vi "Get Scan area.vi"(7 "Inspection data":T1, 8 "error in (no error)":errorcluster, 11 "Programming Data":T12) -> (0 "error out":errorcluster, 2 "Panel size Y":dbl, 3 "Panel Size X":dbl)   [LabVIEW 2013, in "Manipulate IPF.lvlib"]
uses:
  Manipulate IPF.lvlib
  type_def/files.ctl
  3013/code/Modules/Inspection/Data/Panel_class/type_def/Config File data.ctl
  3013/code/Modules/Inspection/type_def/Pos and Rot.ctl
  3013/code/Modules/Inspection/Data/PCB_class/type_def/PCB Params.ctl
  3013/code/Modules/Inspection/Data/Panel_class/type_def/BarCode Params.ctl
  3013/code/Modules/Barcode Reader/type_def/id.ctl
  3013/code/Modules/GUI/GUI_5/subPanels/edit/type_def/data.ctl
  3013/code/Modules/Configuration/type_def/Scan Params.ctl
  3013/code/Modules/Configuration/type_def/Profile Resolution.ctl
  3013/code/Modules/Preprocess Data/type_def/direction.ctl
  3013/code/Modules/Inspection/Data/Panel_class/type_def/inspection data.ctl
  3013/code/Modules/Inspection/type_def/Range Limits.ctl
  type_def/Initial scan size increase.ctl
  <vilib>/Analysis/coordinate.llb/2D Cartesian Coordinate Rotation (Array).vi
  <vilib>/Analysis/coordinate.llb/2D Cartesian Coordinate Shift (Array).vi
  <vilib>/Utility/file.llb/Read From Spreadsheet File (DBL).vi
  <vilib>/Analysis/NI_AALPro.lvlib
  3013/code/Modules/Inspection/Inspection.lvlib
  3013/code/Modules/Inspection/Data/PCB_class/PCB.lvclass
  3013/code/Modules/Barcode Reader/Barcode Reader.lvlib
  3013/code/Modules/Inspection/Data/Panel_class/Panel.lvclass
  a3Di APG.lvlib
  3013/code/Modules/Configuration/Config.lvlib
  3013/code/Modules/Preprocess Data/PreProcess.lvlib
  3013/code/Modules/GUI/GUI_5/subPanels/edit/edit.lvlib
panel:
  out "dbg XY Graph":cluster{"X Out":dbl[], "Y Out":dbl[]}[](graph)
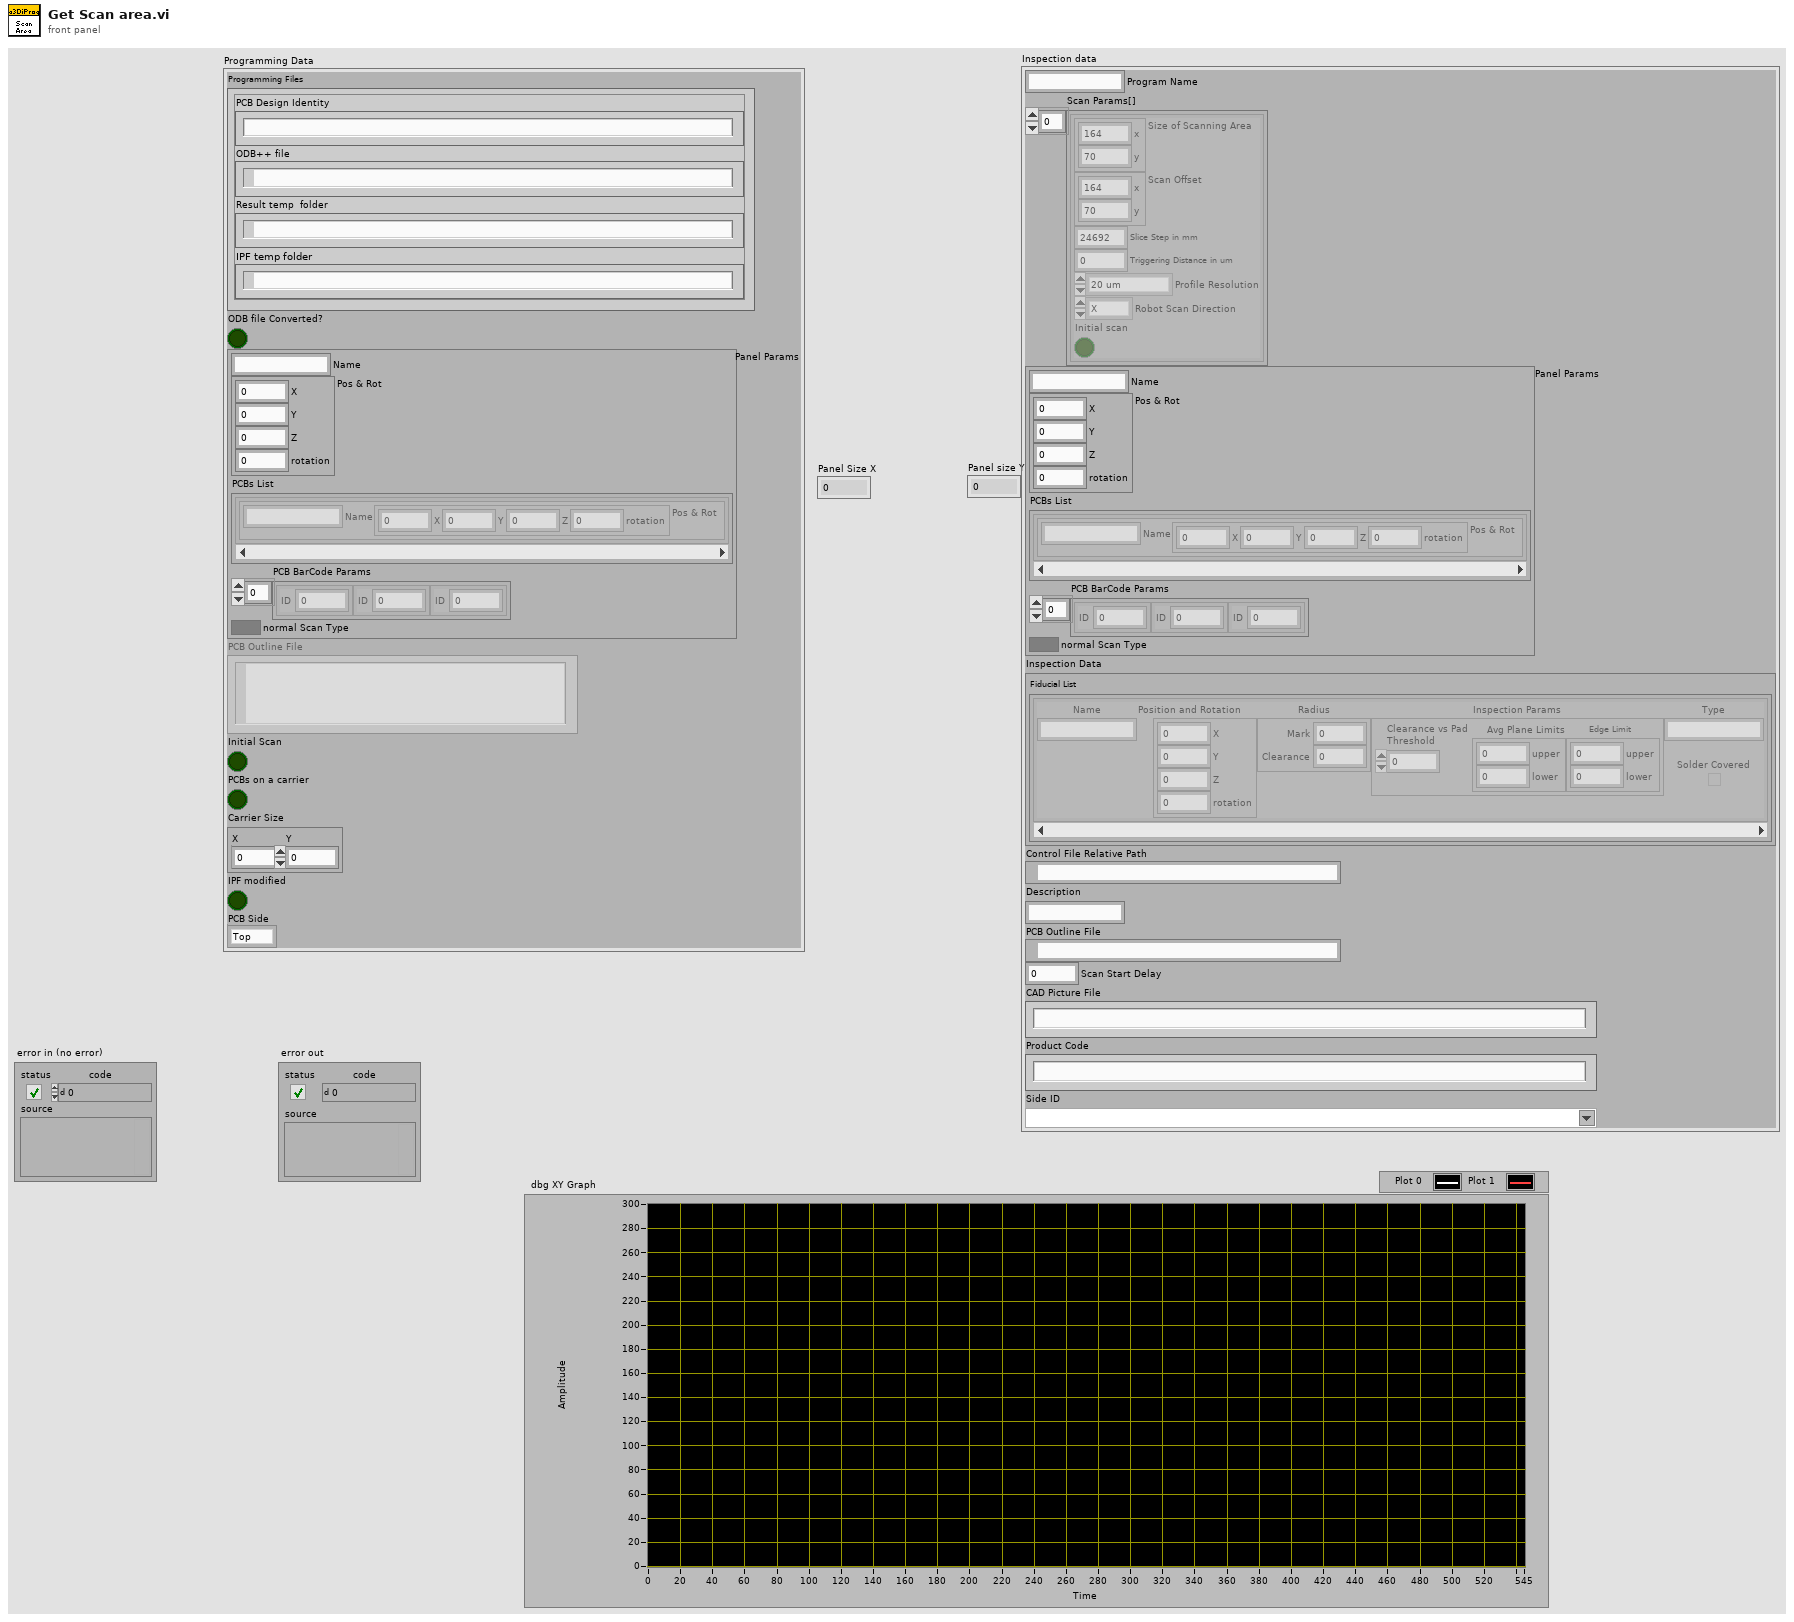
[diagram p1: front panel]
types:
  T1 = typedef "GUI.lvlib/subPanel.lvlib/edit.lvlib/data.ctl" = cluster{"Program Name":string, "Scan Params[]":T2[], "Panel Params":T5, "Inspection Data":T10, "Control File Relative Path":path, "Description":string, "PCB Outline File":path, "Scan Start Delay":dbl, "CAD Picture File":string, "Product Code":string, "Side ID":string}
  T2 = typedef "Config.lvlib/Scan Params.ctl" = cluster{"Size of Scanning Area":cluster{"x":dbl, "y":dbl}, "Scan Offset":cluster{"x":dbl, "y":dbl}, "Slice Step in mm":dbl, "Triggering Distance in mm":dbl, "Triggering Distance in um":dbl, "Profile Resolution":T3, "Version":string, "Robot Scan Direction":T4, "Initial scan":bool}
  T3 = typedef "Config.lvlib/Profile Resolution.ctl" = enum8{"20 um", "40 um"}
  T4 = typedef "PreProcess.lvlib/direction.ctl" = enum8{"X", "Y"}
  T5 = typedef "Inspection.lvlib/Panel.lvclass/Config File data.ctl" = cluster{"Name":string, "Pos & Rot":T6, "PCBs List":cluster{"PCB Params":T7}[], "PCB BarCode Params":T8[], "Scan Type":bool}
  T6 = typedef "Inspection.lvlib/Pos and Rot.ctl" = cluster{"X":dbl, "Y":dbl, "Z":dbl, "rotation":dbl}
  T7 = typedef "Inspection.lvlib/PCB.lvclass/PCB Params.ctl" = cluster{"Name":string, "Pos & Rot":T6}
  T8 = typedef "Inspection.lvlib/Panel.lvclass/BarCode Params.ctl" = cluster{"ID":T9}
  T9 = typedef "Barcode Reader.lvlib/id.ctl" = u8
  T10 = typedef "Inspection.lvlib/Panel.lvclass/inspection data.ctl" = cluster{"Fiducial List":cluster{"Name":string, "Position and Rotation":T6, "Radius":cluster{"Mark":dbl, "Clearance":dbl}, "Inspection Params":cluster{"Clearance vs Pad\nThreshold":dbl, "Avg Plane Limits":T11, "Edge Limit":T11}, "Type":string, "Solder Covered":bool}[]}
  T11 = typedef "Inspection.lvlib/Range Limits.ctl" = cluster{"upper":sgl, "lower":sgl}
  T12 = typedef "a3Di APG.lvlib/files.ctl" = cluster{"Programming Files":cluster{"PCB Design Identity":string, "ODB++ file":path, "Result temp  folder":path, "IPF temp folder":path}, "ODB file Converted?":bool, "Panel Params":T5, "PCB Outline File":path, "Initial Scan":bool, "PCBs on a carrier":bool, "Carrier Size":cluster{"X":dbl, "Y":dbl}, "IPF modified":bool, "PCB Side":enum16{"Top", "Bottom"}}
  T13 = typedef "Manipulate IPF.lvlib/Initial scan size increase.ctl" = dbl
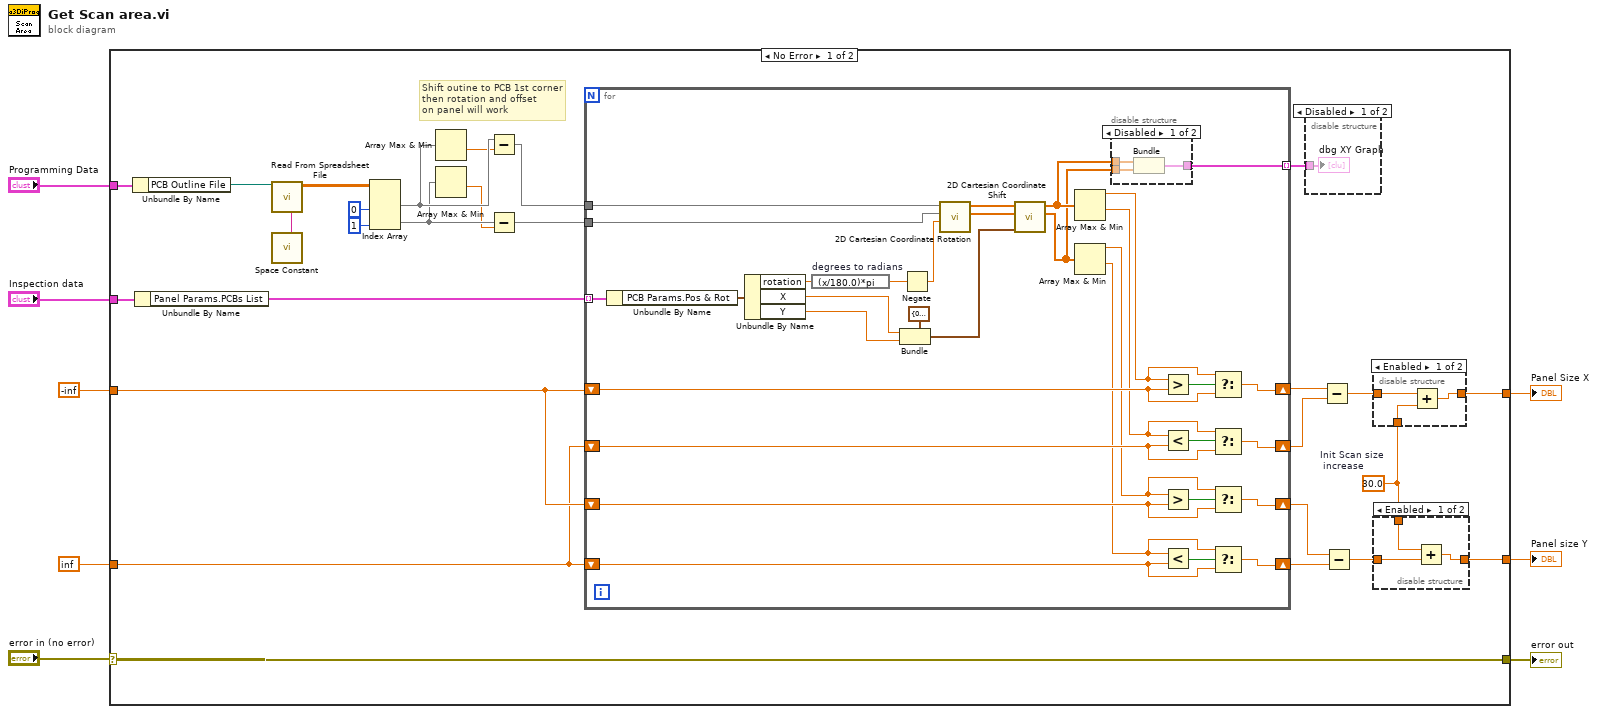
[diagram p0: block diagram]
diagram:
  n1 = case shown="No Error" "error in (no error)" {
    selector: "error in (no error)" -> [w35 w82]
    tunnel: [w35 w82] -> w7
    tunnel: "Programming Data" -> [w34 _]
    tunnel: [w10 w80] -> w5
    tunnel: [w12 w81] -> w6
    tunnel: -inf -> [w26 w81]
    tunnel: inf -> [w25 w80]
    tunnel: "Inspection data" -> [w22 _]
    frame No Error {
      w9 = T13 30.0  # Init Scan size  increase
      # "Shift outine to PCB 1st corner\nthen rotation and offset\non panel will work"
      n2 = Unbundle By Name(w34) -> ("PCB Outline File"=w23:path)
      n3 = Unbundle By Name(w22) -> ("Panel Params.PCBs List"=w21:cluster{"PCB Params":T7}[])
      n4 = call <vilib>:"Space Constant.vi"() -> ("String"=w24:string)
      n5 = call-poly <vilib>:"Read From Spreadsheet File.vi"("delimiter (\\t)"=w24, "file path (dialog if empty)"=w23) -> ("all rows"=w31:dbl[][])  [unwired: 5 in, 4 out]
      n6 = Index Array(array=w31, index (col) #1=0 ("disabled index (col)"), index (col) #2=1 ("index (col)")) -> (element #1=w19:dbl[], element #2=w17:dbl[])  [unwired: 2 in]
      n7 = Array Max & Min(array=w19) -> (min value=w15:dbl)  [unwired: 3 out]
      n8 = Array Max & Min(array=w17) -> (min value=w14:dbl)  [unwired: 3 out]
      n9 = Subtract(x=w19, y=w15) -> (x-y=w18:dbl[])
      n10 = Subtract(x=w17, y=w14) -> (x-y=w16:dbl[])
      n11 = for {
        tunnel: w21 -> [w76] mode=indexing
        tunnel: w18 -> [w68]
        tunnel: w16 -> [w67]
        shift-right: [w64] -> w30
        shift-left: w26 -> [w62]
        shift-right: [w61] -> w28
        shift-left: w26 -> [w60]
        shift-right: [w59] -> w29
        shift-left: w25 -> [w56]
        shift-right: [w55] -> w27
        shift-left: w25 -> [w53]
        tunnel: [w49] -> w20 mode=indexing
        n12 = Unbundle By Name(w76) -> ("PCB Params.Pos & Rot"=w69:T6)
        n13 = Unbundle By Name(w69) -> ("rotation"=w75:dbl, "X"=w72:dbl, "Y"=w71:dbl)
        n14 = expression code="(x/180.0)*pi" "degrees to radians"(w75) -> (w74:dbl)
        n15 = Bundle(cluster=cluster{"dx":dbl, "dy":dbl} {"dx"=0.0, "dy"=0.0} ("shift"), "dx"=w72, "dy"=w71) -> (w70:cluster{"dx":dbl, "dy":dbl})
        n16 = Negate(x=w74) -> (-x=w48:dbl)
        n17 = call-poly <vilib>:"2D Cartesian Coordinate Rotation.vi"("theta"=w48, "Y"=w67, "X"=w68) -> ("Y Out"=w46:dbl[], "X Out"=w47:dbl[])  [unwired: 6 in, 1 out]
        n18 = call-poly <vilib>:"2D Cartesian Coordinate Shift.vi"("shift"=w70, "Y"=w46, "X"=w47) -> ("Y Out"=w50:dbl[], "X Out"=w51:dbl[])  [unwired: 6 in, 1 out]
        n19 = Array Max & Min(array=w51) -> (max value=w65:dbl, min value=w57:dbl)  [unwired: 2 out]
        n20 = Array Max & Min(array=w50) -> (max value=w45:dbl, min value=w52:dbl)  [unwired: 2 out]
        n21 = disable-structure shown="Disabled" {
          disable-tunnel: w51 -> [w79 _]
          disable-tunnel: w50 -> [w78 _]
          disable-tunnel: [w77 _] -> w49
          frame Disabled {
            n22 = Bundle("X Out"=w79, "Y Out"=w78) -> (w77:cluster{"X Out":dbl[], "Y Out":dbl[]})  [unwired: 1 in]
          }
          frame Enabled {
          }
        }
        n23 = Greater?(x=w65, y=w62) -> (0:w66:bool)
        n24 = Less?(x=w57, y=w56) -> (x < y?=w58:bool)
        n25 = Greater?(x=w45, y=w60) -> (0:w63:bool)
        n26 = Less?(x=w52, y=w53) -> (x < y?=w54:bool)
        n27 = Select(t=w65, s=w66, f=w62) -> (s? t:f=w64:dbl)
        n28 = Select(t=w57, s=w58, f=w56) -> (s? t:f=w59:dbl)
        n29 = Select(t=w45, s=w63, f=w60) -> (s? t:f=w61:dbl)
        n30 = Select(t=w52, s=w54, f=w53) -> (s? t:f=w55:dbl)
      }
      n31 = disable-structure shown="Disabled" {
        disable-tunnel: w20 -> [w44 _]
        frame Disabled {
          "dbg XY Graph" <- w44
        }
        frame Enabled {
        }
      }
      n32 = Subtract(x=w30, y=w29) -> (x-y=w13:dbl)
      n33 = Subtract(x=w28, y=w27) -> (x-y=w11:dbl)
      n34 = disable-structure shown="Enabled" {
        disable-tunnel: w13 -> [w42 w43]
        disable-tunnel: [w41 w43] -> w12
        disable-tunnel: w9 -> [w40 _]
        frame Enabled {
          n35 = Add(x=w42, y=w40) -> (x+y=w41:T13)
        }
        frame Disabled {
        }
      }
      n36 = disable-structure shown="Enabled" {
        disable-tunnel: w11 -> [w36 w39]
        disable-tunnel: [w38 w39] -> w10
        disable-tunnel: w9 -> [w37 _]
        frame Enabled {
          n37 = Add(x=w37, y=w36) -> (x+y=w38:T13)
        }
        frame Disabled {
        }
      }
    }
    frame Error {
    }
  }
  "error out" <- w7
  "Panel Size X" <- w6
  "Panel size Y" <- w5
